vi "Tach RPM FPGA.vi"() -> ()   [LabVIEW 2019]
uses:
  <vilib>/eio/EIONode/EIONode.xnode
  <vilib>/rvi/eio/common/nirviEmuTemplateMethod_errors.vi
panel:
  out "ConnectorA/DIO0":bool
  out "Tach State":enum16{"Check Threshold", "Bounce Time"}(ring)
  out "Tach Period (uSec/pulse)":u32
  in  "Slope":enum16{"falling", "rising"}(ring)
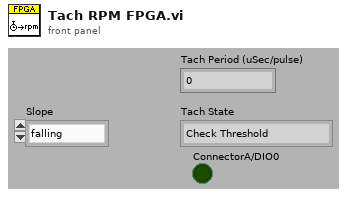
[diagram p1: front panel]
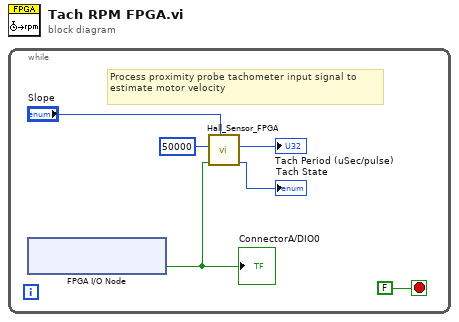
[diagram p0: block diagram]
diagram:
  n1 = while {
    stop <- FALSE stop-if-true
    # "Process proximity probe tachometer input signal to estimate motor velocity"
    n2 = xnode "FPGA I/O Node"() -> ("ConnectorA/DIO0"=w3:bool)  [unwired: 1 in, 1 out]
    "ConnectorA/DIO0" <- w3
    n3 = call "Hall_Sensor_FPGA.vi"("Slope"="Slope", "Hall Sensor"=w3, "Bounce time (uSec)"=u32 50000) -> ("State Out"=→"Tach State":enum16{"Check Threshold", "Bounce Time"}, "Tach Period (uSec/pulse)"=→"Tach Period (uSec/pulse)":u32)  [unwired: 7 in]
  }
